vi "ReadPostAnaly.vi"(9 "shot number":string="123", 10 "Scan":string="Scan043_", 11 "folder path":path) -> (3 "output cluster":cluster{dbl[], dbl[]}[](graph))   [LabVIEW 2020]
uses:
  <vilib>/Utility/file.llb/Read From Spreadsheet File (string).vi
panel:
  out "error IO 2":errorcluster
  in  "error IO":errorcluster
  # "E:\\scan043\\lowE\\Scan043_LESpec_123.txt"
  # "E:\\scan043\\midE\\Scan043_MEDiv_004.txt"
  # "E:\\scan043\\highE\\Scan043_HESpec_067.txt"
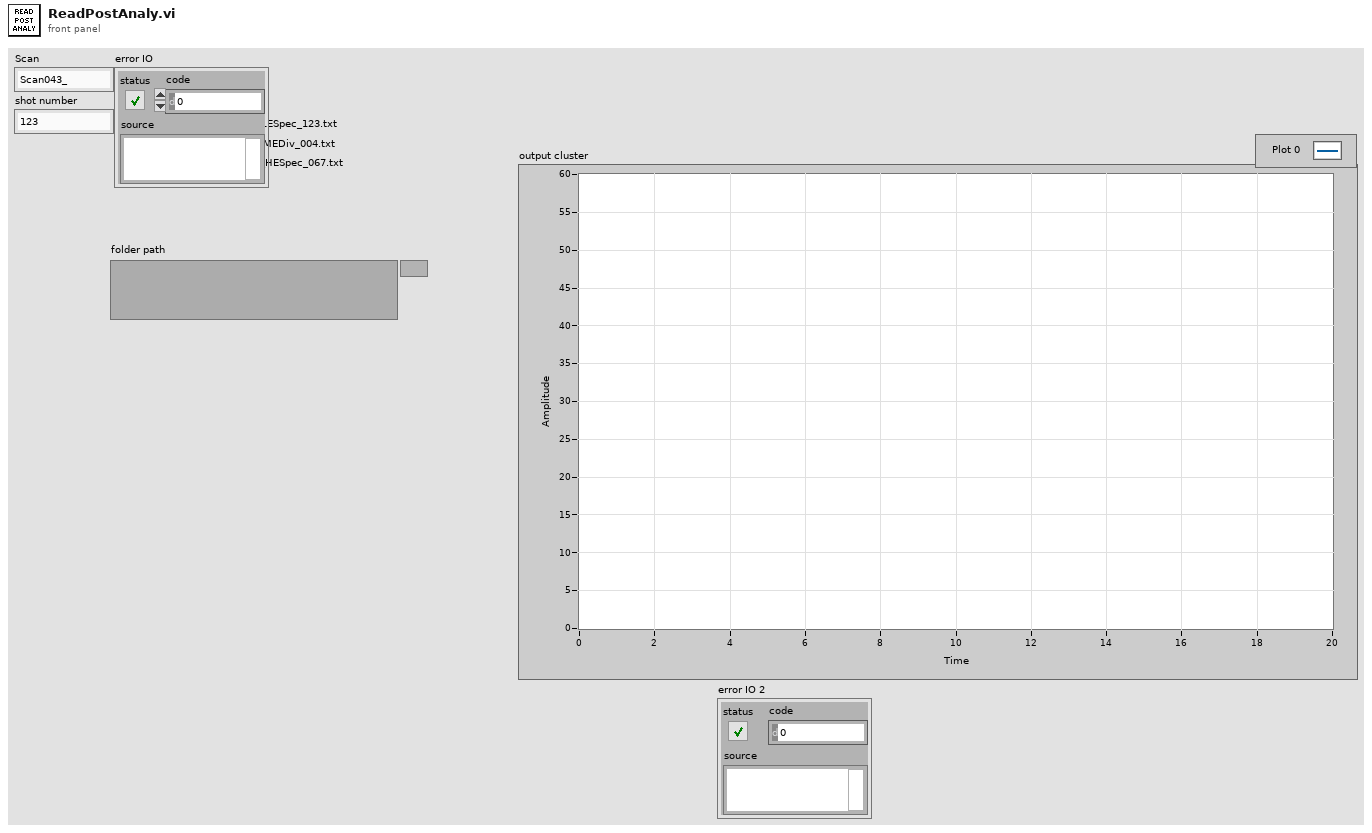
[diagram p1: front panel]
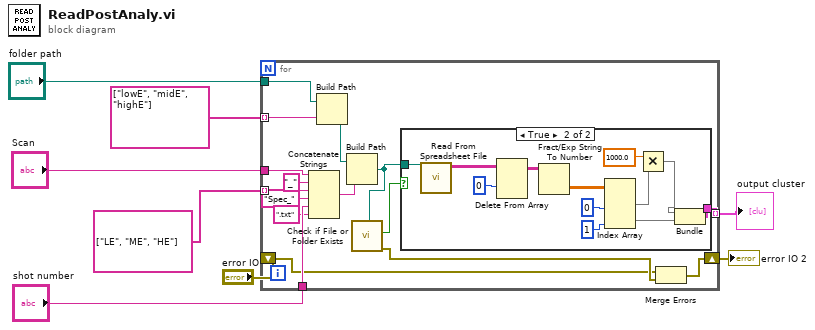
[diagram p0: block diagram]
diagram:
  n1 = for {
    tunnel: "folder path" -> [w24]
    tunnel: string[] ["lowE", "midE", "highE"] -> [w23] mode=indexing
    tunnel: "Scan" -> [w15]
    tunnel: string[] ["LE", "ME", "HE"] -> [w21] mode=indexing
    tunnel: "shot number" -> [w19]
    tunnel: [w16] -> w3 mode=indexing
    shift-right: [w10] -> w1
    shift-left: "error IO" -> [w9]
    n2 = Concatenate Strings(w15, "_" ("string"), w21, "Spec_" ("string"), w19, ".txt" ("string")) -> (w17:string)
    n3 = Build Path(base path=w24, name or relative path=w23) -> (appended path=w22:path)
    n4 = Build Path(base path=w22, name or relative path=w17) -> (appended path=w13:path)
    n5 = call <vilib>:"Check if File or Folder Exists.vi"("path"=w13) -> ("error out"=w11:errorcluster, "file or folder exists?"=w12:bool)  [unwired: 8 in, 1 out]
    n6 = case shown="True" w12 {
      tunnel: [_ w29] -> w16
      tunnel: w13 -> [_ w25]
      frame False {
      }
      frame True {
        n7 = call-poly <vilib>:"Read From Spreadsheet File.vi"("file path (dialog if empty)"=w25) -> ("all rows"=w31:string[][])  [unwired: 6 in, 4 out]
        n8 = Delete From Array(array=w31, index (row)=0) -> (array with subset deleted=w33:string[][])  [unwired: 2 in, 1 out]
        n9 = Fract/Exp String To Number(string=w33) -> (number=w30:dbl[][])  [unwired: 3 in, 1 out]
        n10 = Index Array(array=w30, index (col) #1=0 ("disabled index (col)"), index (col) #2=1 ("disabled index (col)")) -> (element #1=w28:dbl[], element #2=w36:dbl[])  [unwired: 2 in]
        n11 = Multiply(x=1000.0, y=w28) -> (x*y=w26:dbl[])
        n12 = Bundle(w26, w36) -> (w29:cluster{dbl[], dbl[]})  [unwired: 1 in]
      }
    }
    n13 = Merge Errors(w9, w11) -> (w10:errorcluster)
  }
  "output cluster" <- w3
  "error IO 2" <- w1
